vi "Configure Resolution and Video Bandwidth.vi"(8 "error in (no error)":errorcluster, 9 "VBW [Hz]":dbl, 10 "RBW [Hz]":dbl, 11 "SA-ESA in":refnum<class "SA-ESA.lvclass">) -> (0 "error out":errorcluster, 3 "SA-ESA out":refnum<class "SA-ESA.lvclass">)   [LabVIEW 2020, in "SA-ESA.lvclass"]
uses:
  SA-ESA.lvclass
  C:/Sandbox/RF Bench/Source Code/WiSpry Test Framework/Instruments/Instrument.lvclass
  C:/Sandbox/RF Bench/Source Code/WiSpry Test Framework/Instruments/Spectrum Analyzer/Spectrum Analyzer.lvclass
  Instrument.lvclass/Instrument.ctl
  Spectrum Analyzer.lvclass/Spectrum Analyzer.ctl
  Instrument.lvclass
  Spectrum Analyzer.lvclass
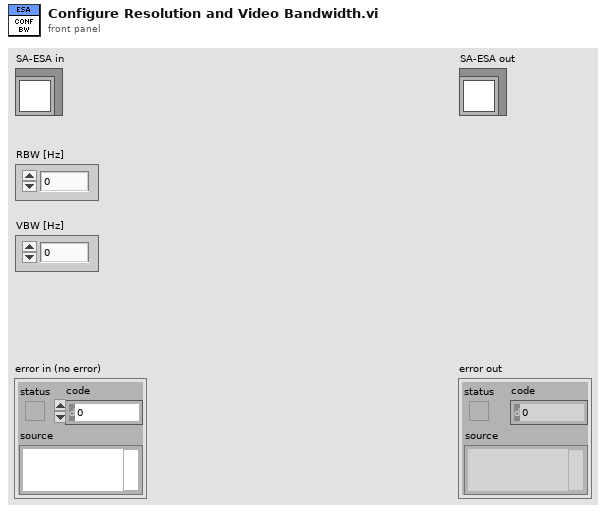
[diagram p1: front panel]
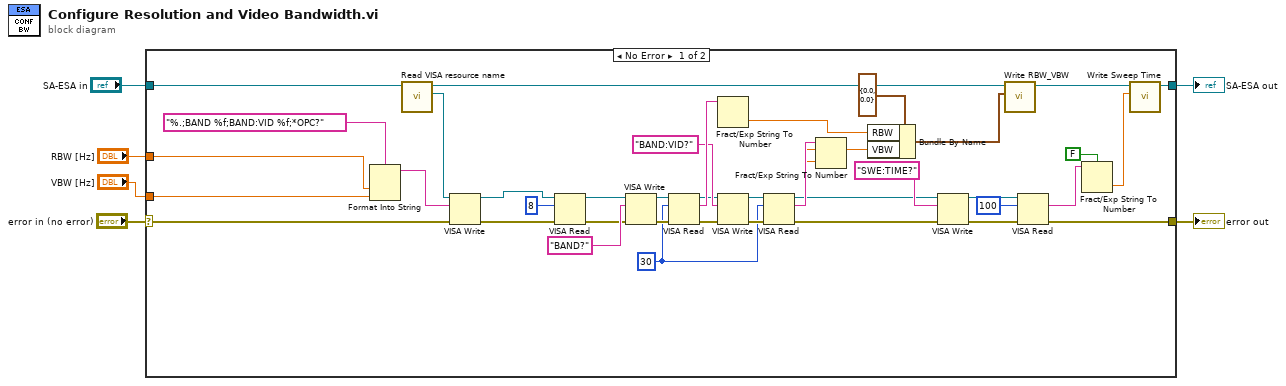
[diagram p0: block diagram]
diagram:
  n1 = case shown="No Error" "error in (no error)" {
    selector: "error in (no error)" -> [w40 w47]
    tunnel: "SA-ESA in" -> [w43 w48]
    tunnel: "RBW [Hz]" -> [w45 _]
    tunnel: "VBW [Hz]" -> [w44 _]
    tunnel: [w32 w47] -> w1
    tunnel: [w31 w48] -> w2
    frame No Error {
      w20 = u32 30 ("byte count")
      n2 = Format Into String(format string="%.;BAND %f;BAND:VID %f;*OPC?", w45, w44) -> (resulting string=w41:string)  [unwired: 2 in, 1 out]
      n3 = call "Read VISA resource name.vi"("Instrument in"=w43) -> ("VISA resource name"=w42:refnum<visa-resource-name>, "Instrument out"=w19:refnum<class "SA-ESA.lvclass">)  [unwired: 9 in]
      n4 = VISA Write(VISA resource name=w42, write buffer=w41, error in (no error)=w40) -> (VISA resource name out=w9:refnum<visa-resource-name>, error out=w12:errorcluster)  [unwired: 1 out]
      n5 = VISA Read(VISA resource name=w9, byte count=u32 8, error in (no error)=w12) -> (VISA resource name out=w10:refnum<visa-resource-name>, error out=w11:errorcluster)  [unwired: 2 out]
      n6 = VISA Write(VISA resource name=w10, write buffer="BAND?", error in (no error)=w11) -> (VISA resource name out=w28:refnum<visa-resource-name>, error out=w29:errorcluster)  [unwired: 1 out]
      n7 = VISA Read(VISA resource name=w28, byte count=w20, error in (no error)=w29) -> (VISA resource name out=w22:refnum<visa-resource-name>, read buffer=w27:string, error out=w21:errorcluster)  [unwired: 1 out]
      n8 = Fract/Exp String To Number(string=w27) -> (number=w16:dbl)  [unwired: 3 in, 1 out]
      n9 = VISA Write(VISA resource name=w22, write buffer="BAND:VID?", error in (no error)=w21) -> (VISA resource name out=w25:refnum<visa-resource-name>, error out=w24:errorcluster)  [unwired: 1 out]
      n10 = VISA Read(VISA resource name=w25, byte count=w20, error in (no error)=w24) -> (VISA resource name out=w7:refnum<visa-resource-name>, read buffer=w26:string, error out=w8:errorcluster)  [unwired: 1 out]
      n11 = Fract/Exp String To Number(string=w26) -> (number=w15:dbl)  [unwired: 3 in, 1 out]
      n12 = Bundle By Name(cluster=cluster{"RBW":dbl, "VBW":dbl} {"RBW"=0.0, "VBW"=0.0} ("RBW/VBW"), "RBW"=w16, "VBW"=w15) -> (w14:cluster{"RBW":dbl, "VBW":dbl})
      n13 = VISA Write(VISA resource name=w7, write buffer="SWE:TIME?", error in (no error)=w8) -> (VISA resource name out=w37:refnum<visa-resource-name>, error out=w38:errorcluster)  [unwired: 1 out]
      n14 = call "Write RBW_VBW.vi"("RBW/VBW"=w14, "Spectrum Analyzer in"=w19) -> ("Spectrum Analyzer out"=w18:refnum<class "SA-ESA.lvclass">)  [unwired: 9 in]
      n15 = VISA Read(VISA resource name=w37, byte count=u32 100, error in (no error)=w38) -> (read buffer=w35:string, error out=w32:errorcluster)  [unwired: 2 out]
      n16 = Fract/Exp String To Number(use system decimal point (T)=FALSE, string=w35) -> (number=w33:dbl)  [unwired: 2 in, 1 out]
      n17 = call "Write Sweep Time.vi"("Sweep Time"=w33, "Spectrum Analyzer in"=w18) -> ("Spectrum Analyzer out"=w31:refnum<class "SA-ESA.lvclass">)  [unwired: 9 in]
    }
    frame Error {
    }
  }
  "error out" <- w1
  "SA-ESA out" <- w2
